vi "PH_4_Pos_Selector.get Position.vi"(0 "i ref in":refnum<vi>, 5 "error in (no error)":errorcluster) -> (14 "i ref out":refnum<vi>, 19 "error out":errorcluster)   [LabVIEW 2014, in "PH_4_Pos_Selector.lvlib"]
doc: "This VI gets the Position and sets - related to that - GUI elements."
uses:
  PH_4_Pos_Selector.lvlib
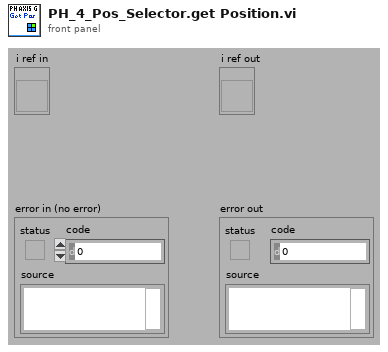
[diagram p1: front panel]
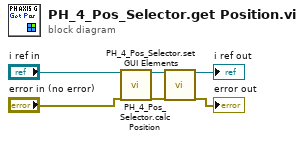
[diagram p0: block diagram]
diagram:
  n1 = call "PH_4_Pos_Selector.calc Position.vi"("i ref in"="i ref in", "error in (no error)"="error in (no error)") -> ("i ref out"=w3:refnum<vi>, "error out"=w5:errorcluster)  [unwired: 16 in]
  n2 = call "PH_4_Pos_Selector.set GUI Elements.vi"("i ref in"=w3, "error in (no error)"=w5) -> ("i ref out"=→"i ref out":refnum<vi>, "error out"=→"error out":errorcluster)  [unwired: 16 in]
